vi "Read State UART.vi"(8 "error in (no error)":errorcluster, 11 "GiaoTiepUART in":refnum<class "GiaoTiepUART.lvclass">) -> (0 "error out":errorcluster, 2 "STATEUART":T1, 3 "GiaoTiepUART out":refnum<class "GiaoTiepUART.lvclass">)   [LabVIEW 2017, in "LibraryGcode.lvlib" / "GiaoTiepUART.lvclass"]
uses:
  GiaoTiepUART.lvclass
  StateMachine_UART.ctl
  GiaoTiepUART.lvclass/GiaoTiepUART.ctl
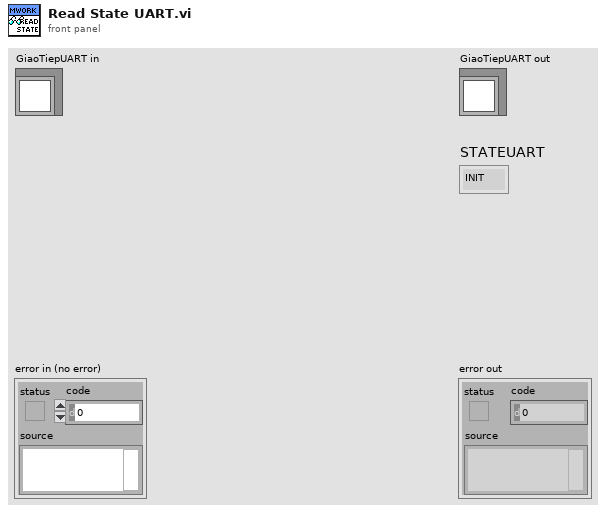
[diagram p1: front panel]
types:
  T1 = typedef "LibraryGcode.lvlib/GiaoTiepUART.lvclass/StateMachine_UART.ctl" = enum16{"INIT", "WRITE", "READ", "CHECKDATA", "IDLE", "STOP"}
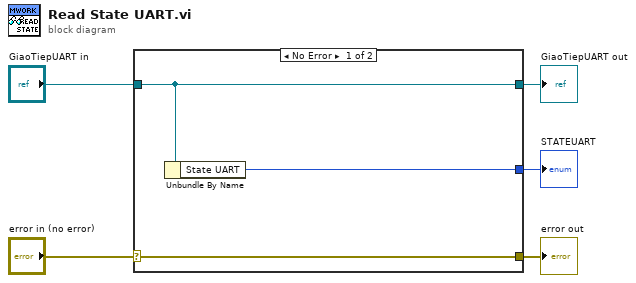
[diagram p0: block diagram]
diagram:
  n1 = case shown="No Error" "error in (no error)" {
    selector: "error in (no error)" -> [w8 w9]
    tunnel: [w8 w9] -> w4
    tunnel: [w7 w10] -> w2
    tunnel: "GiaoTiepUART in" -> [w7 w10]
    tunnel: [w6 _] -> w1
    frame No Error {
      n2 = Unbundle By Name(w7) -> ("State UART"=w6:T1)
    }
    frame Error {
    }
  }
  "error out" <- w4
  "GiaoTiepUART out" <- w2
  "STATEUART" <- w1
